vi "main (1).vi"() -> ()   [LabVIEW 2023]
uses:
  CONTROLS/states.ctl
panel:
  out "Meldung":string
  out "Enum":T1
  in  "stop":bool
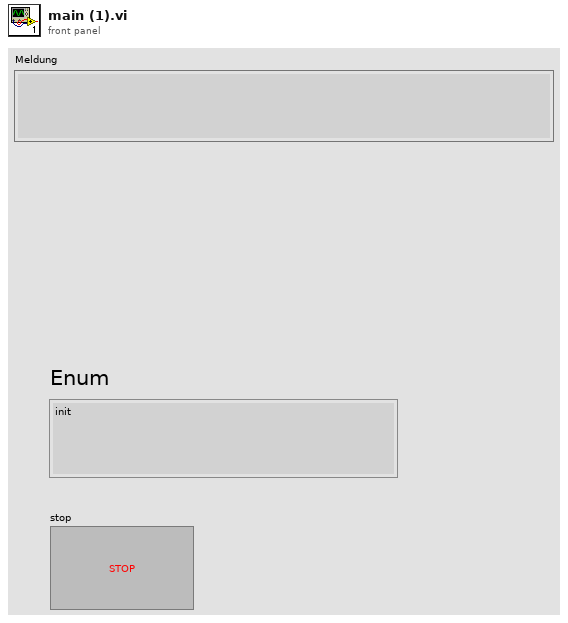
[diagram p1: front panel]
types:
  T1 = typedef "states.ctl" = enum16{"init", "read", "write", "Kundeneingabe", "Betonauswahl", "Bezahlprozeß", "Rechnung", "Zudaten mit Gewichtmessung", "Stop"}
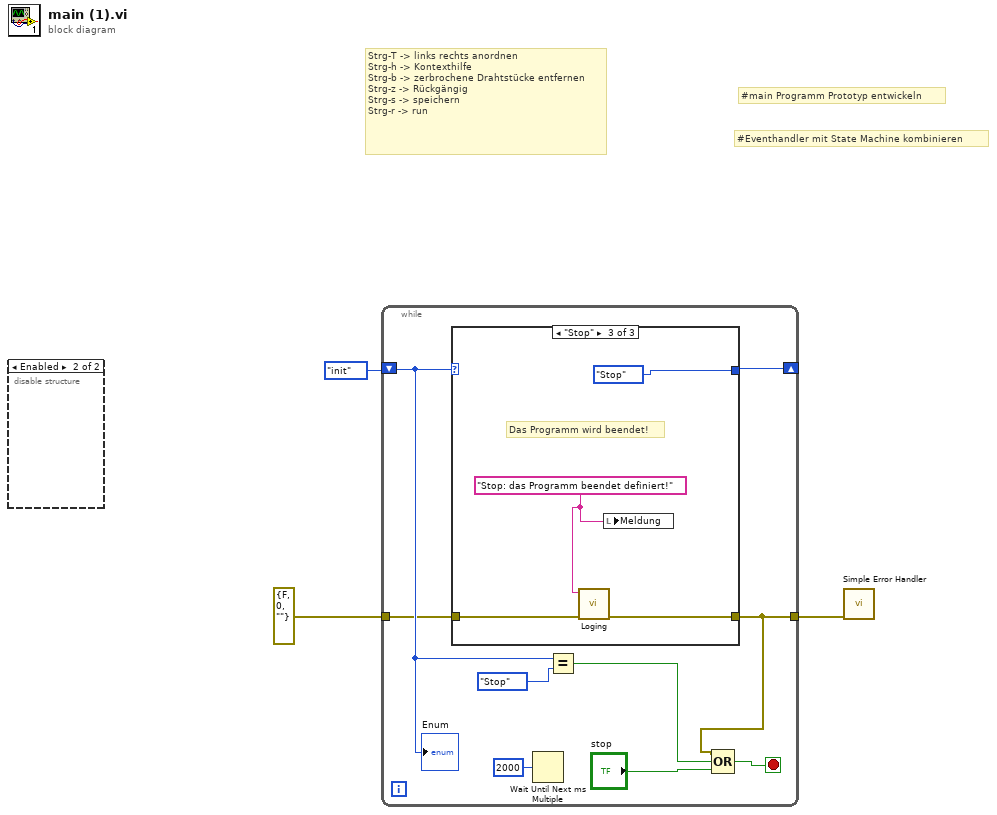
[diagram p0: block diagram]
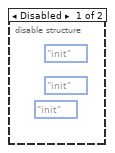
[diagram p2: hidden frame]
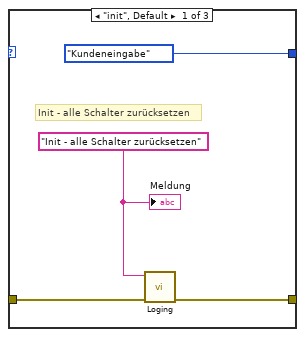
[diagram p3: hidden frame]
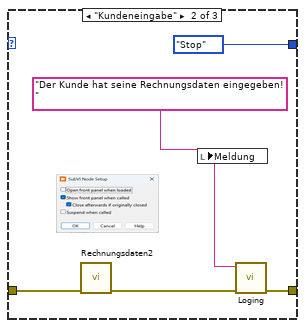
[diagram p4: hidden frame]
diagram:
  # "#Eventhandler mit State Machine kombinieren"
  # "#main Programm Prototyp entwickeln"
  # "Strg-T -> links rechts anordnen\nStrg-h -> Kontexthilfe\nStrg-b -> zerbrochene Drahtstücke entfernen\nStrg-z -> Rückgängig\nStrg-s -> speichern\nStrg-r -> run"
  n1 = disable-structure shown="Enabled" {
    frame Disabled {
      (unwired) states."init"
      (unwired) states."init"
      (unwired) states."init"
    }
    frame Enabled {
    }
  }
  n2 = while {
    shift-right: [w12] -> _
    shift-left: states."init" -> [w10]
    tunnel: errorcluster {"status"=FALSE, "code"=0, "source"=""} ("error in") -> [w5]
    tunnel: [w4] -> w2
    stop <- w7 stop-if-true
    n3 = case shown="\"Stop\"" w10 {
      tunnel: [states."Kundeneingabe" states."Stop" states."Stop"] -> w12
      tunnel: w5 -> [w14 w18 w23]
      tunnel: [w13 w19 w22] -> w4
      frame "init", Default {
        w15 = "Init - alle Schalter zurücksetzen" ("Meldung")
        # "Init - alle Schalter zurücksetzen"
        n4 = call "Loging.vi"("error in"=w14, "log"=w15) -> ("error out"=w13:errorcluster)  [unwired: 9 in]
        "Meldung" <- w15
      }
      frame "Kundeneingabe" {
        w20 = "Der Kunde hat seine Rechnungsdaten eingegeben!   " ("Meldung")
        n5 = call "Rechnungsdaten2.vi"("error in (no error)"=w18) -> ("error out"=w17:errorcluster)  [unwired: 10 in]
        n6 = local write "Meldung"(w20) -> ()
        n7 = call "Loging.vi"("error in"=w17, "log"=w20) -> ("error out"=w19:errorcluster)  [unwired: 9 in]
      }
      frame "Stop" {
        w24 = "Stop: das Programm beendet definiert!" ("Meldung")
        # "Das Programm wird beendet!"
        n8 = call "Loging.vi"("error in"=w23, "log"=w24) -> ("error out"=w22:errorcluster)  [unwired: 9 in]
        n9 = local write "Meldung"(w24) -> ()
      }
    }
    n10 = Wait Until Next ms Multiple(millisecond multiple=u32 2000) -> ()  [unwired: 1 out]
    n11 = Equal?(x=w10, y=states."Stop") -> (x = y?=w9:bool)
    n12 = Compound Arithmetic op=OR(w4, w9, "stop") -> (w7:bool)
    "Enum" <- w10
  }
  n13 = call <vilib>:"Simple Error Handler.vi"("error in (no error)"=w2) -> ()  [unwired: 4 in, 5 out]
